vi "SMUSine.vi"() -> ()   [LabVIEW 2023]
uses:
  <instrlib>/niDCPower/nidcpower.llb/niDCPower Sequence Attribute Type.ctl
  <instrlib>/niDCPower/nidcpower.llb/niDCPower Source Mode.ctl
  <instrlib>/niDCPower/nidcpower.llb/niDCPower Output Function.ctl
  <instrlib>/niDCPower/nidcpower.llb/niDCPower Create Advanced Sequence Step With Channels.vi
panel:
  in  "?":enum32{"Standard Transients", "Custom"}(tab)
  in  "Source:Transient Response":i32(ring)=1041 items=["Slow"=1041, "Normal"=1038, "Fast"=1039, "Custom"=1042]
  in  "Gain Bandwidth":dbl=5000.0
  in  "Pole-Zero Ratio":dbl=0.16
  in  "Compensation Frequency":dbl=50000.0
  out "Stimulus In":cluster{dbl, dbl}[](graph)
  out "Apperature Time":dbl format="%#_6p"
  out "SMU Voltage Out":cluster{dbl, dbl}[](graph)
  in  "Amount of Sine Swings":i32
  in  "Fixed Source Delay of":dbl format="%#_6p"
  in  "Samples per Sine":u16
  in  "Frequency":dbl format="%#_6p"
  in  "Amplitude":dbl
  in  "DC offset":dbl
  out "error out":errorcluster
  in  "resource name":refnum<k15>
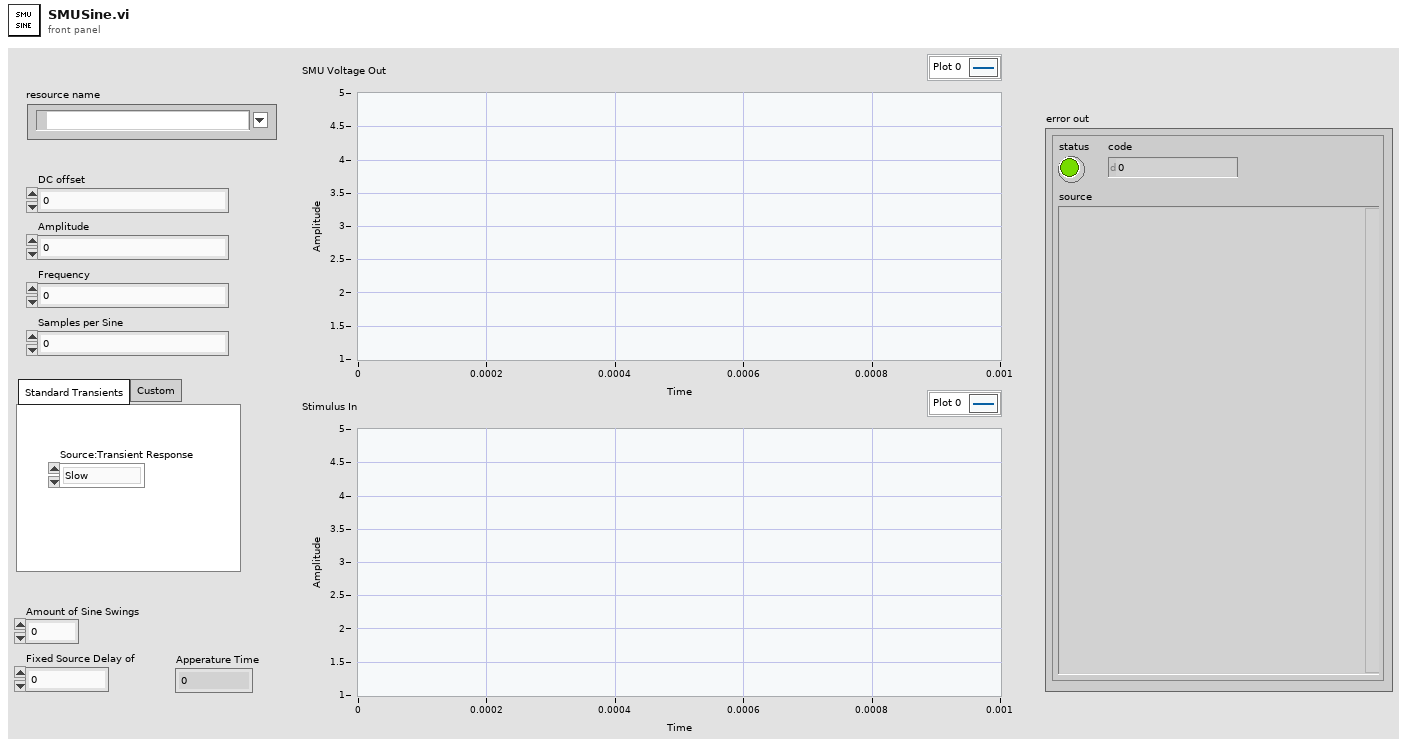
[diagram p1: front panel]
types:
  T1 = typedef "niDCPower Output Function.ctl" = i32
  T2 = typedef "niDCPower Source Mode.ctl" = i32
  T3 = typedef "niDCPower Sequence Attribute Type.ctl" = i32
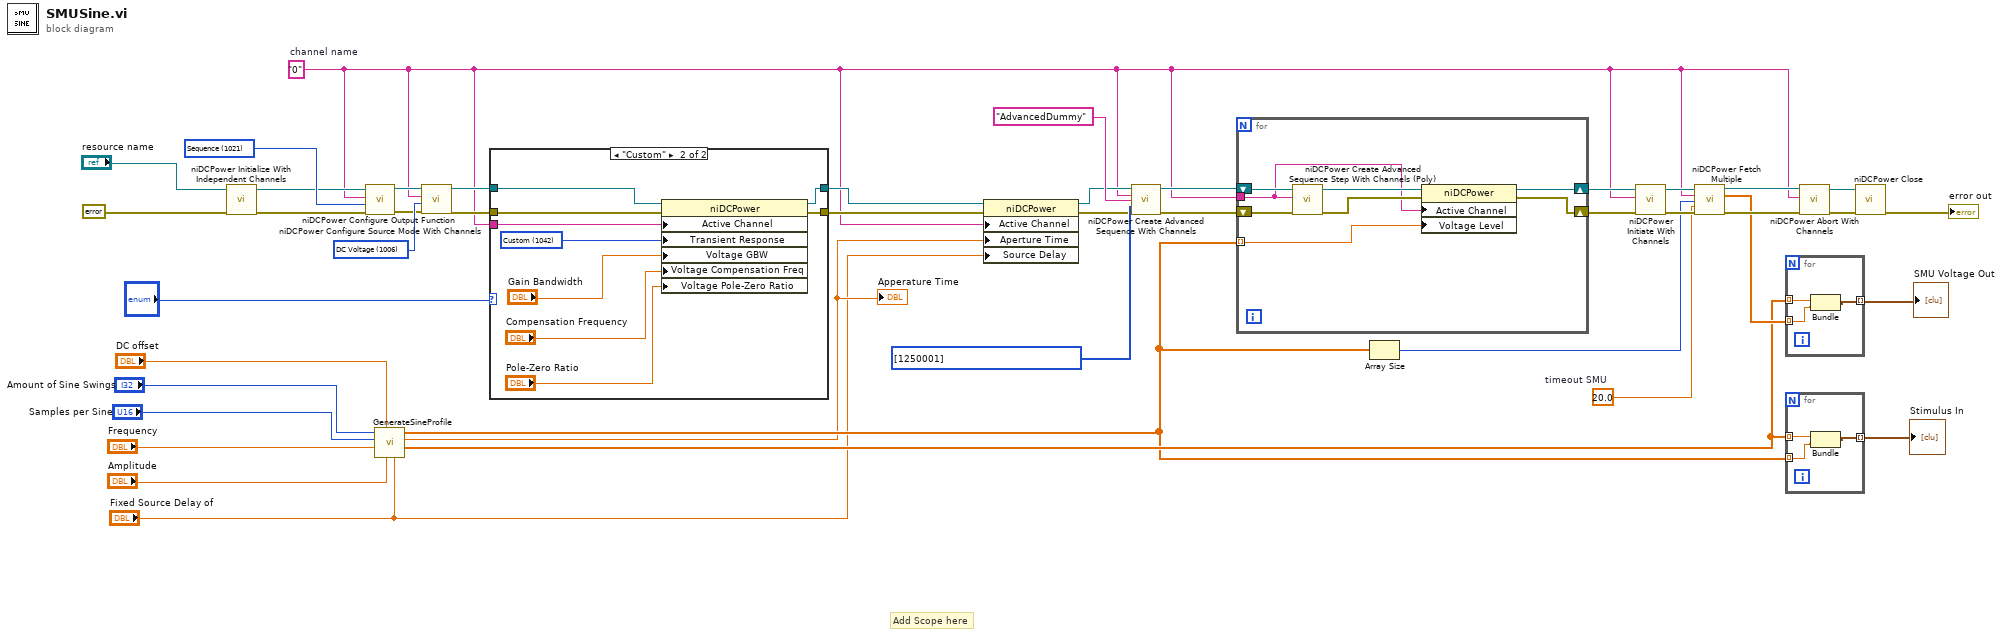
[diagram p0: block diagram]
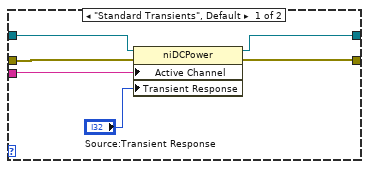
[diagram p2: hidden frame]
diagram:
  w12 = 20.0  # timeout SMU
  w27 = T1 1006 items=["DC Voltage"=1006, "DC Current"=1007, "Pulse Voltage"=1049, "Pulse Current"=1050] ("output function")
  w30 = T2 1021 items=["Single Point"=1020, "Sequence"=1021] ("source mode")
  w32 = T3[] [1250001] items=["Source -> Output Function"=1150008, "Source -> Output Enabled"=1250006, "Source -> Output Resistance"=1150061, "Source -> Transient Response"=1150062, "Source -> Custom Transient Response -> Voltage Gain Bandwidth"=1150067, "Source -> Custom Transient Response -> Voltage Compensation Frequency"=1150068, "Source -> Custom Transient Response -> Voltage Pole-Zero Ratio"=1150069, "Source -> Custom Transient Response -> Current Gain Bandwidth"=1150070, "Source -> Custom Transient Response -> Current Compensation Frequency"=1150071, "Source -> Custom Transient Response -> Current Pole-Zero Ratio"=1150072, "Source -> DC Voltage -> Voltage Level"=1250001, "Source -> DC Voltage -> Voltage Level Range"=1150005, "Source -> DC Voltage -> Current Limit"=1250005, "Source -> DC Voltage -> Current Limit High"=1150187, "Source -> DC Voltage -> Current Limit Low"=1150188, "Source -> DC Voltage -> Current Limit Range"=1150004, "Source -> DC Current -> Current Level"=1150009, "Source -> DC Current -> Current Level Range"=1150011, "Source -> DC Current -> Voltage Limit"=1150010, "Source -> DC Current -> Voltage Limit High"=1150185, "Source -> DC Current -> Voltage Limit Low"=1150186, "Source -> DC Current -> Voltage Limit Range"=1150012, "Source -> DC Current -> Current Level Slew Rate -> Rising"=1150343, "Source -> DC Current -> Current Level Slew Rate -> Falling"=1150344, "Source -> Pulse Voltage -> Pulse Voltage Level"=1150080, "Source -> Pulse Voltage -> Pulse Bias Voltage Level"=1150082, "Source -> Pulse Voltage -> Pulse Voltage Level Range"=1150084, "Source -> Pulse Voltage -> Pulse Current Limit"=1150081, "Source -> Pulse Voltage -> Pulse Current Limit High"=1150193, "Source -> Pulse Voltage -> Pulse Current Limit Low"=1150194, "Source -> Pulse Voltage -> Pulse Bias Current Limit"=1150083, "Source -> Pulse Voltage -> Pulse Bias Current Limit High"=1150195, "Source -> Pulse Voltage -> Pulse Bias Current Limit Low"=1150196, "Source -> Pulse Voltage -> Pulse Current Limit Range"=1150085, "Source -> Pulse Current -> Pulse Current Level"=1150086, "Source -> Pulse Current -> Pulse Bias Current Level"=1150088, "Source -> Pulse Current -> Pulse Current Level Range"=1150090, "Source -> Pulse Current -> Pulse Voltage Limit"=1150087, "Source -> Pulse Current -> Pulse Voltage Limit High"=1150189, "Source -> Pulse Current -> Pulse Voltage Limit Low"=1150190, "Source -> Pulse Current -> Pulse Bias Voltage Limit"=1150089, "Source -> Pulse Current -> Pulse Bias Voltage Limit High"=1150191, "Source -> Pulse Current -> Pulse Bias Voltage Limit Low"=1150192, "Source -> Pulse Current -> Pulse Voltage Limit Range"=1150091, "Source -> Advanced -> Source Delay"=1150051, "Source -> Advanced -> Pulse Bias Delay"=1150092, "Source -> Advanced -> Pulse On Time"=1150093, "Source -> Advanced -> Pulse Off Time"=1150094, "Source -> Advanced -> OVP Enabled"=1250002, "Source -> Advanced -> OVP Limit"=1250003, "Source -> Advanced -> Compliance Limit Symmetry"=1150184, "Source -> Advanced -> Sequence Step Delta Time"=1150198, "Source -> Advanced -> Conduction Voltage -> Mode"=1150350, "Source -> Advanced -> Conduction Voltage -> On Threshold"=1150351, "Source -> Advanced -> Conduction Voltage -> Off Threshold"=1150352, "Measurement -> Sense"=1150013, "Measurement -> Aperture Time"=1150058, "Measurement -> Measure Record Length"=1150063, "Measurement -> Advanced -> DC Noise Rejection"=1150066, "Measurement -> Autorange"=1150244, "Measurement -> Advanced -> Autorange Behavior"=1150245, "Measurement -> Advanced -> Autorange Aperture Time Mode"=1150246, "Measurement -> Advanced -> Autorange Minimum Aperture Time"=1150247, "Measurement -> Advanced -> Autorange Minimum Aperture Time Units"=1150248, "Measurement -> Advanced -> Autorange Minimum Current Range"=1150255, "Measurement -> Advanced -> Autorange Minimum Voltage Range"=1150256, "Measurement -> Advanced -> Autorange Threshold Mode"=1150257, "Measurement -> Advanced -> Autorange Maximum Delay After Range Change"=1150322, "LCR -> Instrument Mode"=1150208, "LCR -> Source Delay Mode"=1150315, "LCR -> Measurement Time"=1150218, "LCR -> Custom Measurement Time"=1150258, "LCR -> AC Stimulus -> Function"=1150209, "LCR -> AC Stimulus -> Frequency"=1150210, "LCR -> AC Stimulus -> Voltage Amplitude"=1150211, "LCR -> AC Stimulus -> Current Amplitude"=1150212, "LCR -> AC Stimulus -> Advanced -> Voltage Range"=1150265, "LCR -> AC Stimulus -> Advanced -> Current Range"=1150267, "LCR -> AC Stimulus -> Advanced -> Source Aperture Time"=1150349, "LCR -> DC Bias -> Source"=1150213, "LCR -> DC Bias -> Voltage Level"=1150214, "LCR -> DC Bias -> Current Level"=1150215, "LCR -> DC Bias -> Advanced -> Voltage Range"=1150266, "LCR -> DC Bias -> Advanced -> Current Range"=1150274, "LCR -> DC Bias -> Advanced -> Transient Response"=1150347, "LCR -> Compensation -> Open -> Enabled"=1150220, "LCR -> Compensation -> Open -> Conductance"=1150261, "LCR -> Compensation -> Open -> Susceptance"=1150262, "LCR -> Compensation -> Short -> Enabled"=1150221, "LCR -> Compensation -> Short -> Resistance"=1150263, "LCR -> Compensation -> Short -> Reactance"=1150264, "LCR -> Compensation -> Load -> Enabled"=1150222, "LCR -> Compensation -> Load -> Measured Resistance"=1150268, "LCR -> Compensation -> Load -> Measured Reactance"=1150269, "LCR -> Compensation -> Load -> Actual Resistance"=1150270, "LCR -> Compensation -> Load -> Actual Reactance"=1150271, "LCR -> Impedance Range -> Impedance Range"=1150217, "LCR -> Impedance Range -> Impedance Autorange"=1150216, "LCR -> Impedance Range -> Advanced -> Impedance Range Source"=1150321, "LCR -> Impedance Range -> Advanced -> Load Resistance"=1150318, "LCR -> Impedance Range -> Advanced -> Load Inductance"=1150319, "LCR -> Impedance Range -> Advanced -> Load Capacitance"=1150320] ("advanced sequence properties")
  w4 = "0"  # channel name
  # "Add Scope here"
  n1 = call <instrlib>:"niDCPower Initialize With Independent Channels.vi"("error in (no error)"=errorcluster {"status"=FALSE, "code"=0, "source"=""}, "resource name"="resource name") -> ("error out"=w28:errorcluster, "instrument handle out"=w29:refnum<k15>)  [unwired: 8 in]
  n2 = call <instrlib>:"niDCPower Configure Source Mode With Channels.vi"("error in (no error)"=w28, "source mode"=w30, "channel name"=w4, "instrument handle"=w29) -> ("error out"=w25:errorcluster, "instrument handle out"=w26:refnum<k15>)  [unwired: 6 in]
  n3 = call "GenerateSineProfile.vi"("Fixed Source Delay of"="Fixed Source Delay of", "Amplitude"="Amplitude", "DC offset"="DC offset", "Frequency"="Frequency", "Samples per Sine"="Samples per Sine", "Amount of Itterations"="Amount of Sine Swings") -> ("Time to Plot"=w10:dbl[], "Apperature Time"=w3:dbl, "Voltage"=w9:dbl[])  [unwired: 3 in]
  "Apperature Time" <- w3
  n4 = call <instrlib>:"niDCPower Configure Output Function.vi"("error in (no error)"=w25, "output function"=w27, "channel name"=w4, "instrument handle"=w26) -> ("error out"=w19:errorcluster, "instrument handle out"=w18:refnum<k15>)  [unwired: 6 in]
  n5 = case shown="\"Custom\"" "?" {
    tunnel: [w49 w58] -> w7
    tunnel: w19 -> [w46 w57]
    tunnel: w18 -> [w47 w56]
    tunnel: w4 -> [w45 w55]
    tunnel: [w48 w54] -> w8
    frame "Standard Transients", Default {
      n6 = property class="niDCPower"(reference=w47, error in=w46, "Active Channel"=w45, "Transient Response"="Source:Transient Response") -> (reference out=w48:refnum<k15>, error out=w49:errorcluster)
    }
    frame "Custom" {
      w53 = 1042 items=["Slow"=1041, "Normal"=1038, "Fast"=1039, "Custom"=1042] ("Source:Transient Response")
      n7 = property class="niDCPower"(reference=w56, error in=w57, "Active Channel"=w55, "Transient Response"=w53, "Voltage GBW"="Gain Bandwidth", "Voltage Compensation Freq"="Compensation Frequency", "Voltage Pole-Zero Ratio"="Pole-Zero Ratio") -> (reference out=w54:refnum<k15>, error out=w58:errorcluster)
    }
  }
  n8 = property class="niDCPower"(reference=w8, error in=w7, "Active Channel"=w4, "Aperture Time"=w3, "Source Delay"="Fixed Source Delay of") -> (reference out=w6:refnum<k15>, error out=w5:errorcluster)
  n9 = call <instrlib>:"niDCPower Create Advanced Sequence With Channels.vi"("instrument handle"=w6, "channel name"=w4, "sequence name"="AdvancedDummy", "advanced sequence properties"=w32, "error in (no error)"=w5) -> ("instrument handle out"=w20:refnum<k15>, "error out"=w21:errorcluster)  [unwired: 9 in]
  n10 = for {
    tunnel: w4 -> [w60]
    shift-right: [w61] -> w41
    shift-left: w20 -> [w66]
    shift-right: [w62] -> w40
    shift-left: w21 -> [w65]
    tunnel: w9 -> [w59] mode=indexing
    n11 = call-poly <instrlib>:"niDCPower Create Advanced Sequence Step With Channels (Poly).vi"("error in (no error)"=w65, "channel name"=w60, "instrument handle"=w66) -> ("error out"=w64:errorcluster, "instrument handle out"=w63:refnum<k15>)  [unwired: 7 in]
    n12 = property class="niDCPower"(reference=w63, error in=w64, "Active Channel"=w60, "Voltage Level"=w59) -> (reference out=w61:refnum<k15>, error out=w62:errorcluster)
  }
  n13 = Array Size(array=w9) -> (size(s)=w24:i32)
  n14 = call <instrlib>:"niDCPower Initiate With Channels.vi"("error in (no error)"=w40, "channel name"=w4, "instrument handle"=w41) -> ("error out"=w38:errorcluster, "instrument handle out"=w39:refnum<k15>)  [unwired: 7 in]
  n15 = call <instrlib>:"niDCPower Fetch Multiple.vi"("instrument handle"=w39, "channel name"=w4, "count (1)"=w24, "timeout (1.0)"=w12, "error in (no error)"=w38) -> ("instrument handle out"=w43:refnum<k15>, "voltage measurements"=w15:dbl[], "error out"=w42:errorcluster)  [unwired: 5 in, 3 out]
  n16 = for {
    tunnel: w10 -> [w69] mode=indexing
    tunnel: w15 -> [w68] mode=indexing
    tunnel: [w67] -> w14 mode=indexing
    n17 = Bundle(w69, w68) -> (w67:cluster{dbl, dbl})  [unwired: 1 in]
  }
  "SMU Voltage Out" <- w14
  n18 = for {
    tunnel: w10 -> [w72] mode=indexing
    tunnel: w9 -> [w71] mode=indexing
    tunnel: [w70] -> w11 mode=indexing
    n19 = Bundle(w72, w71) -> (w70:cluster{dbl, dbl})  [unwired: 1 in]
  }
  "Stimulus In" <- w11
  n20 = call <instrlib>:"niDCPower Abort With Channels.vi"("error in (no error)"=w42, "channel name"=w4, "instrument handle"=w43) -> ("error out"=w36:errorcluster, "instrument handle out"=w37:refnum<k15>)  [unwired: 7 in]
  n21 = call <instrlib>:"niDCPower Close.vi"("error in (no error)"=w36, "instrument handle"=w37) -> ("error out"=→"error out":errorcluster)  [unwired: 9 in]
